vi "03 Python Node.vi"() -> ()   [LabVIEW 2019]
uses:
  _Subs/OpenDiagram/Open_XControl.xctl
panel:
  out "Volume":dbl
  out "area":dbl
  in  "diameter":dbl=2.0
  in  "OpenDiag":refnum<vi>(xcontrol)
  # "03 Python Node\nThis code shows how to talk to Python Code\n\nInstructions:\n1. Make sure you have Python 3.7 installed on your machine"
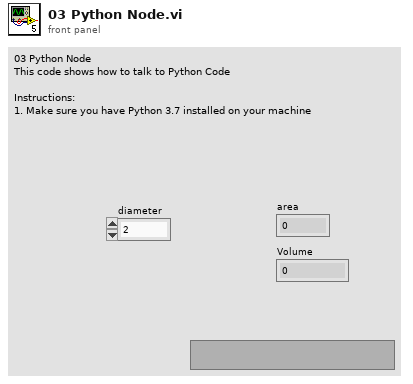
[diagram p1: front panel]
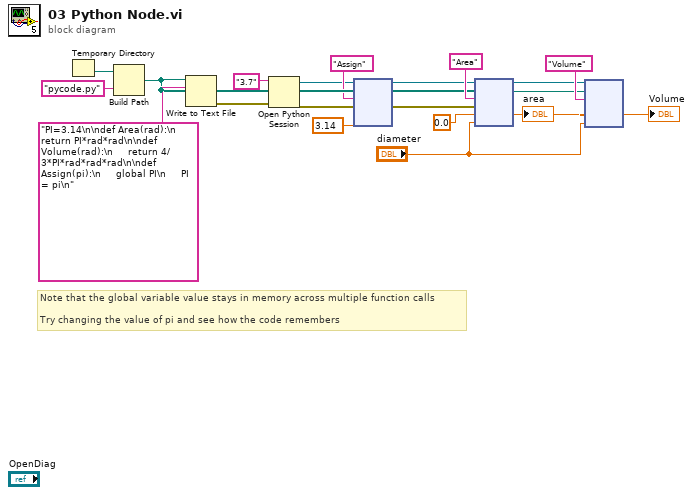
[diagram p0: block diagram]
diagram:
  # "Note that the global variable value stays in memory across multiple function calls\n\nTry changing the value of pi and see how the code remembers"
  n1 = Temporary Directory() -> (w14:path)
  n2 = Build Path(base path=w14, name or relative path="pycode.py") -> (appended path=w5:path)
  n3 = Write to Text File(file (use dialog)=w5, text="PI=3.14\n\ndef Area(rad):\n     return PI*rad*rad\n\ndef Volume(rad):\n     return 4/3*PI*rad*rad*rad\n\ndef Assign(pi):\n     global PI\n     PI = pi\n") -> (error out=w11:errorcluster)  [unwired: 2 in, 2 out]
  n4 = Open Python Session(python version="3.7" ("Python version"), 3:w11) -> (session out=w2:refnum<k35>, error out=w15:errorcluster)  [unwired: 1 in]
  n5 = node(w2, w5, "Assign" ("function name"), 3.14) -> (w1:refnum<k35>)  [unwired: 4 in, 3 out]
  n6 = node(w1, w5, "Area" ("function name"), w15, 0.0, "diameter") -> (w8:refnum<k35>, w6:dbl)  [unwired: 1 in, 3 out]
  "area" <- w6
  n7 = node(w8, w5, "Volume" ("function name"), w6, "diameter") -> (→"Volume":dbl)  [unwired: 2 in, 4 out]
